vi "Create_directory_option.vi"(0 "Filename":path) -> (1 "Path is to existing File":bool, 2 "Path is to existing Directory":bool)   [LabVIEW 2021]
uses:
  Globals/Preference_global.vi
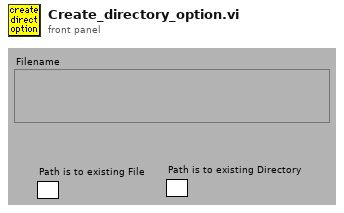
[diagram p1: front panel]
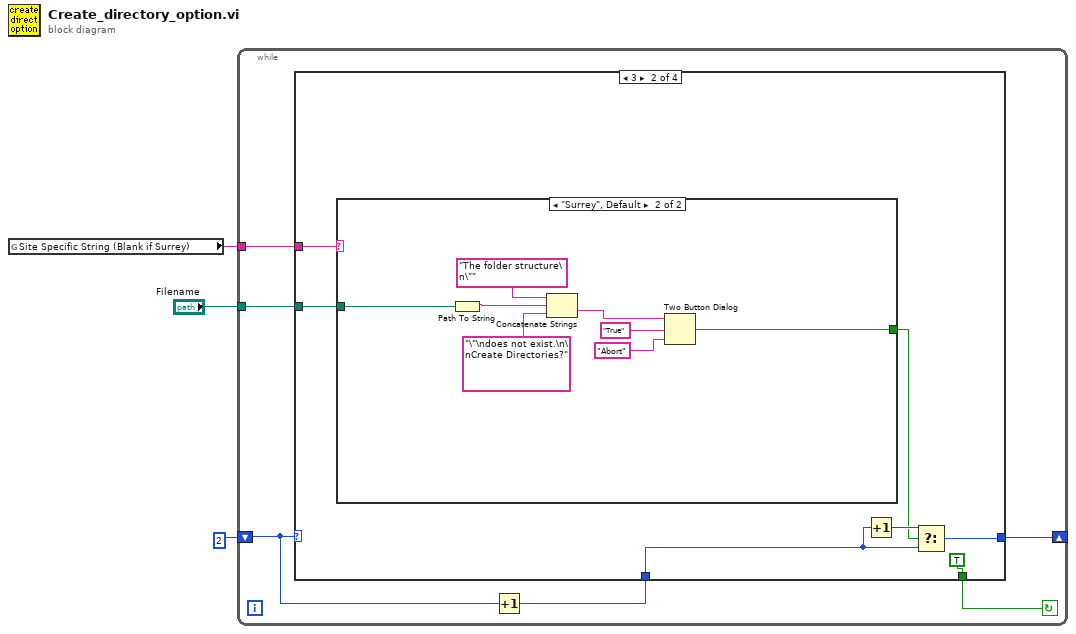
[diagram p0: block diagram]
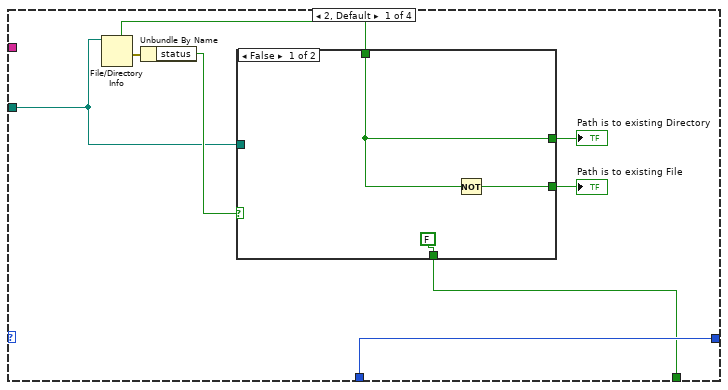
[diagram p2: hidden frame]
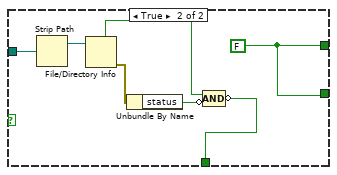
[diagram p3: hidden frame]
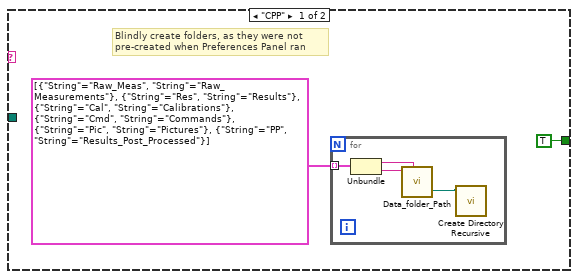
[diagram p4: hidden frame]
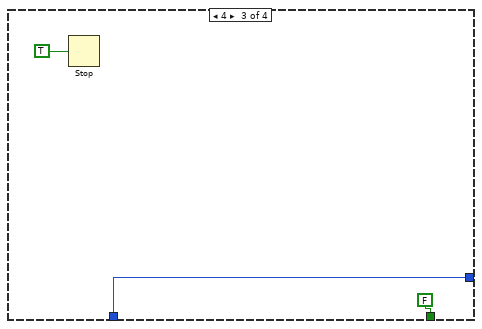
[diagram p5: hidden frame]
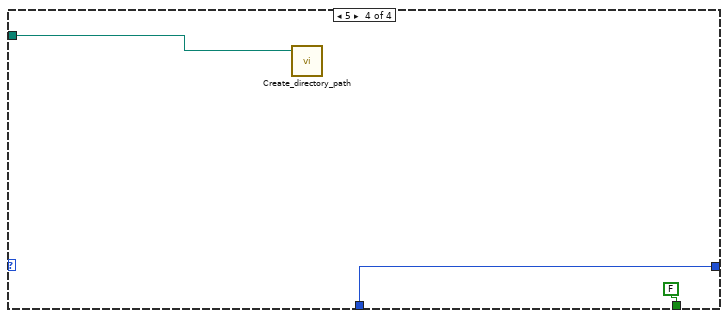
[diagram p6: hidden frame]
diagram:
  n1 = global read "Preference_global.vi" "Site Specific String (Blank if Surrey)"() -> (w1:string)
  n2 = while {
    tunnel: "Filename" -> [w5]
    shift-left: 2 -> [w8]
    shift-right: [w6] -> _
    tunnel: w1 -> [w4]
    stop <- w9 continue-if-true
    n3 = Increment(x=w8) -> (x+1=w7:i32)
    n4 = case shown="3" w8 {
      tunnel: [w10 TRUE ("status") FALSE ("status") FALSE ("status")] -> w9
      tunnel: w7 -> [w17 w32 w49 w54]
      tunnel: [w17 w30 w49 w54] -> w6
      tunnel: w5 -> [w11 w34 _ w52]
      tunnel: w4 -> [_ w28 _ _]
      frame 2, Default {
        n5 = File/Directory Info(path=w11) -> (directory=w13:bool, error out=w16:errorcluster)  [unwired: 1 in, 5 out]
        n6 = Unbundle By Name(w16) -> ("status"=w12:bool)
        n7 = case shown="False" w12 {
          tunnel: [w20 w24] -> w15
          tunnel: [w19 w24] -> w14
          tunnel: w13 -> [w20 _]
          tunnel: w11 -> [_ w26]
          tunnel: [FALSE ("status") w21] -> w10
          frame False {
            n8 = Not(x=w20) -> (.not. x?=w19:bool)
          }
          frame True {
            w24 = FALSE ("Directory exists")
            n9 = Strip Path(path=w26) -> (stripped path=w25:path)  [unwired: 1 out]
            n10 = File/Directory Info(path=w25) -> (directory=w23:bool, error out=w27:errorcluster)  [unwired: 1 in, 5 out]
            n11 = Unbundle By Name(w27) -> ("status"=w22:bool)
            n12 = Compound Arithmetic op=AND(w23, invert w22) -> (invert w21:bool)
          }
        }
        "Path is to existing File" <- w14
        "Path is to existing Directory" <- w15
      }
      frame 3 {
        n13 = case shown="\"Surrey\", Default" w28 {
          tunnel: w34 -> [_ w42]
          tunnel: [TRUE ("T button?") w41] -> w29
          frame "CPP" {
            # "Blindly create folders, as they were not \npre-created when Preferences Panel ran"
            n14 = for {
              tunnel: cluster{"String":string, "String":string}[] [{"String"="Raw_Meas", "String"="Raw_Measurements"}, {"String"="Res", "String"="Results"}, {"String"="Cal", "String"="Calibrations"}, {"String"="Cmd", "String"="Commands"}, {"String"="Pic", "String"="Pictures"}, {"String"="PP", "String"="Results_Post_Processed"}] ("array of clusters") -> [w40] mode=indexing
              n15 = Unbundle(w40) -> ("String"=w39:string, "String"=w38:string)
              n16 = call "Data_folder_Path.vi"("Data Type"=w38, "Short_Name"=w39) -> ("Data Folder"=w37:path)  [unwired: 4 in]
              n17 = call <vilib>:"Create Directory Recursive.vi"("directory"=w37) -> ()  [unwired: 4 in, 3 out]
            }
          }
          frame "Surrey", Default {
            n18 = Path To String(path=w42) -> (string=w48:string)
            n19 = Concatenate Strings("The folder structure\n\"", w48, "\"\ndoes not exist.\n\nCreate Directories?") -> (w45:string)
            n20 = Two Button Dialog(message=w45, 1:"Abort" ("F button name (\"Cancel\")"), 2:"True" ("T button name (\"OK\")")) -> (T button?=w41:bool)
          }
        }
        n21 = Increment(x=w32) -> (x+1=w31:i32)
        n22 = Select(t=w31, s=w29, f=w32) -> (s? t:f=w30:i32)
      }
      frame 4 {
        n23 = Stop(stop? (T)=TRUE) -> ()
      }
      frame 5 {
        n24 = call "Create_directory_path.vi"("Path name"=w52) -> ()  [unwired: 2 in, 2 out]
      }
    }
  }
